vi "Meas Result Update View.vi"(8 "error in":errorcluster, 10 "gui refs":T15, 11 "meas":T3 {"swp cfg"."f list"."bias" format="%#_3p"; "swp cfg"."f list"."level" format="%#_3p"; "swp cfg"."f list"."fs [Hz]" format="%#_5p"; "swp cfg"."f list"."time [s]" format="%#_3p"; "swp cfg"."f list"."f/fs" format="%#_3p"; "swp cfg"."f list"."periods" format="%#_3f"; "swp cfg"."f list"."f [Hz]" format="%#_5p"}) -> (0 "error out":errorcluster)   [LabVIEW 2013]
doc: "Update results view."
uses:
  Meas Result GUI References.ctl
  Meas Result Freq Format.ctl
  meas session.ctl
  Meas Sweep Config.ctl
  Meas Freq Info.ctl
  meas_swp_mode.ctl
  meas_sweep_flist_mode.ctl
  bridge/Bridge Session.ctl
  bridge/Bridge Type.ctl
  drivers/TWM client/TWM Session.ctl
  drivers/TWM client/TWM parameters.ctl
  source/Source Session.ctl
  source/Source Type.ctl
  drivers/AFG3101C/AFG3101C Session.ctl
  Meas Results.ctl
  bridge/Bridge Frequency Readings Data.ctl
  Meas Result Major Format.ctl
  Meas Result Deviation Format.ctl
  varilib/varilib.lvlib
panel:
  in  "mjr dev fmt":T1 caption="Enum"
  in  "mjr fmt":T2
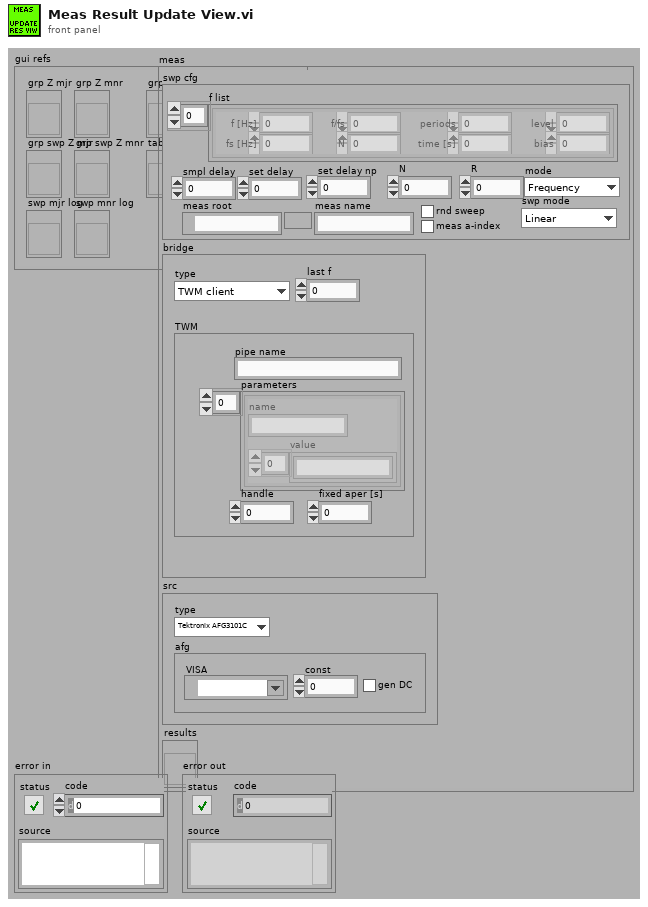
[diagram p1: front panel]
types:
  T1 = typedef "Meas Result Deviation Format.ctl" = enum16{"abs", "%", "ppm"}
  T2 = typedef "Meas Result Major Format.ctl" = enum16{"%_5p", "%_6p", "%_7p", "%_8p", "%_5f", "%_6f", "%_7f", "%_8f"}
  T3 = typedef "meas session.ctl" = cluster{"swp cfg":T4, "bridge":T8, "src":T12, "results":refnum<vi>}
  T4 = typedef "Meas Sweep Config.ctl" = cluster{"N":i32, "R":i32, "f list":T5[], "smpl delay":dbl, "set delay":dbl, "set delay np":dbl, "meas root":path, "meas name":string, "meas a-index":bool, "rnd sweep":bool, "mode":T6, "swp mode":T7}
  T5 = typedef "Meas Freq Info.ctl" = cluster{"f [Hz]":dbl, "periods":dbl, "f/fs":dbl, "time [s]":dbl, "fs [Hz]":dbl, "N":i32, "level":dbl, "bias":dbl}
  T6 = typedef "meas_swp_mode.ctl" = enum16{"Frequency", "Level", "Bias"}
  T7 = typedef "meas_sweep_flist_mode.ctl" = enum16{"Linear", "Log10"}
  T8 = typedef "Bridge Session.ctl" = cluster{"type":T9, "TWM":T10, "last f":dbl}
  T9 = typedef "Bridge Type.ctl" = enum16{"TWM client", "dummy"}
  T10 = typedef "TWM Session.ctl" = cluster{"pipe name":string, "parameters":T11[], "handle":i32, "fixed aper [s]":dbl}
  T11 = typedef "TWM parameters.ctl" = cluster{"name":string, "value":string[]}
  T12 = typedef "Source Session.ctl" = cluster{"type":T13, "afg":T14}
  T13 = typedef "Source Type.ctl" = enum16{"Tektronix AFG3101C", "dummy"}
  T14 = typedef "AFG3101C Session.ctl" = cluster{"VISA":refnum<visa-resource-name>, "const":dbl, "gen DC":bool}
  T15 = typedef "Meas Result GUI References.ctl" = cluster{"grp Z mjr":refnum<vi>, "grp Z mnr":refnum<vi>, "grp swp Z mjr":refnum<vi>, "grp swp Z mnr":refnum<vi>, "swp mjr log":refnum<vi>, "swp mnr log":refnum<vi>, "grp ref":refnum<vi>, "tab swp":refnum<vi>, "mjr fmt":refnum<vi>, "mnr fmt":refnum<vi>, "mjr dev fmt":refnum<vi>, "mnr dev fmt":refnum<vi>, "res frq fmt":refnum<vi>}
  T16 = typedef "Meas Results.ctl" = cluster{"freqs":T17[], "locked":bool, "last fid":i32, "modified":bool, "mjr name":string, "mnr name":string}
  T17 = typedef "Bridge Frequency Readings Data.ctl" = cluster{"Udut":dbl[], "Iref":dbl[], "Udc":dbl[], "Idc":dbl[], "mjr":dbl[], "mnr":dbl[], "n":i32, "f [Hz]":dbl}
  T18 = typedef "Meas Results Sweep Data.ctl" = cluster{"Udut":dbl[], "Iref":dbl[], "Udc":dbl[], "Idc":dbl[], "mjr":dbl[], "mnr":dbl[], "f [Hz]":dbl[]}
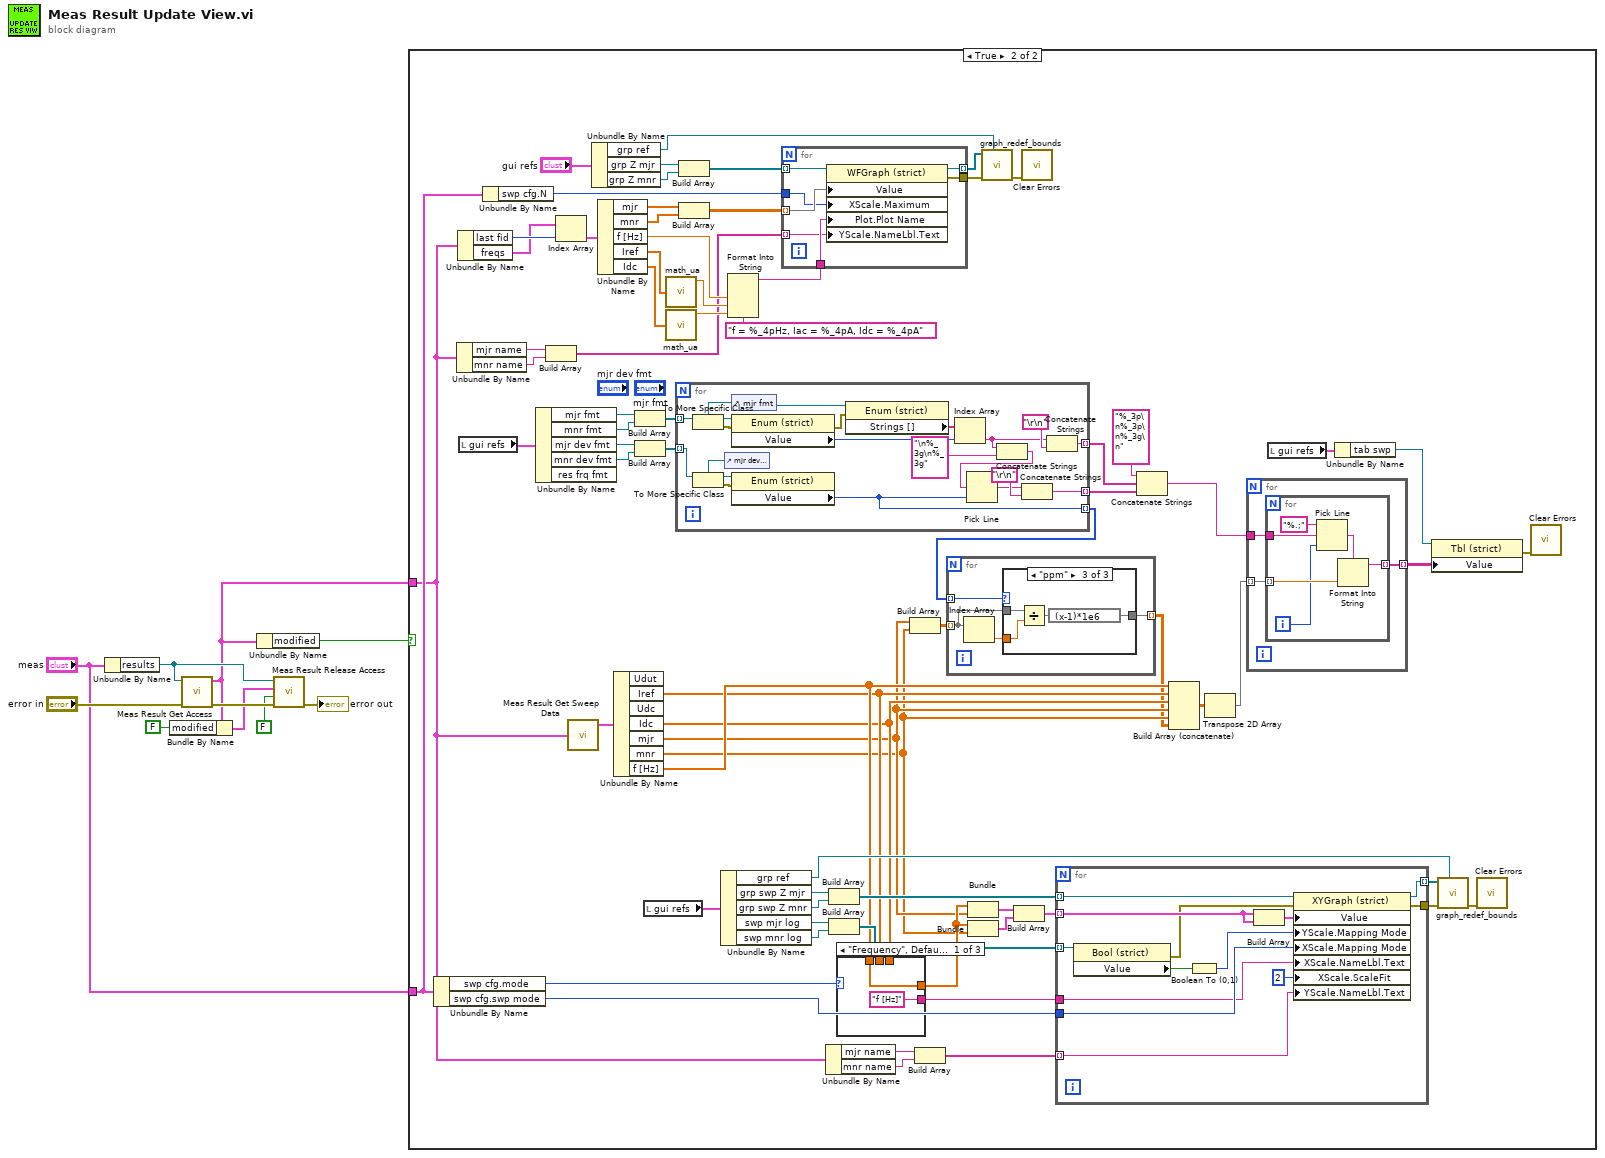
[diagram p0: block diagram]
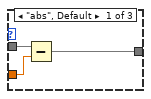
[diagram p3: hidden frame]
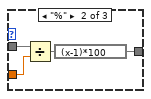
[diagram p4: hidden frame]
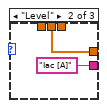
[diagram p5: hidden frame]
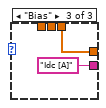
[diagram p6: hidden frame]
diagram:
  n1 = Unbundle By Name("meas") -> ("results"=w9:refnum<vi>)
  n2 = call "Meas Result Get Access.vi"("error in"="error in", "results ref"=w9) -> ("error out"=w10:errorcluster, "results data"=w2:T16)  [unwired: 8 in]
  n3 = Bundle By Name(cluster=w2, "modified"=FALSE) -> (w5:T16)
  n4 = Unbundle By Name(w2) -> ("modified"=w6:bool)
  n5 = call "Meas Result Release Access.vi"("error in"=w10, "Release only (True)"=FALSE, "results data in"=w5, "results ref"=w9) -> ("error out"=→"error out":errorcluster)  [unwired: 7 in]
  n6 = case shown="True" w6 {
    tunnel: w2 -> [_ w12]
    tunnel: "meas" -> [_ w46]
    frame False {
    }
    frame True {
      n7 = Unbundle By Name(w46) -> ("swp cfg.mode"=w67:T6, "swp cfg.swp mode"=w62:T7)
      n8 = Unbundle By Name(w12) -> ("mjr name"=w17:string, "mnr name"=w16:string)
      n9 = Unbundle By Name(w12) -> ("last fid"=w83:i32, "freqs"=w82:T17[])
      n10 = local read "gui refs"() -> (w33:T15)
      n11 = Unbundle By Name(w46) -> ("swp cfg.N"=w45:i32)
      n12 = Unbundle By Name(w33) -> ("mjr fmt"=w32:refnum<vi>, "mnr fmt"=w31:refnum<vi>, "mjr dev fmt"=w29:refnum<vi>, "mnr dev fmt"=w28:refnum<vi>)  [unwired: 1 out]
      n13 = Build Array(w17, w16) -> (w15:string[])
      n14 = Index Array(array=w82, index=w83) -> (element=w78:T17)
      n15 = call "Meas Result Get Sweep Data.vi"("result"=w12) -> ("data"=w37:T18)  [unwired: 2 out]
      n16 = Unbundle By Name("gui refs") -> ("grp ref"=w55:refnum<vi>, "grp Z mjr"=w81:refnum<vi>, "grp Z mnr"=w80:refnum<vi>)
      n17 = Unbundle By Name(w78) -> ("mjr"=w77:dbl[], "mnr"=w76:dbl[], "f [Hz]"=w39:dbl, "Iref"=w41:dbl[], "Idc"=w42:dbl[])
      n18 = Unbundle By Name(w37) -> ("Iref"=w35:dbl[], "Idc"=w34:dbl[], "mjr"=w22:dbl[], "mnr"=w21:dbl[], "f [Hz]"=w36:dbl[])  [unwired: 2 out]
      n19 = Build Array(w32, w31) -> (w30:refnum<vi>[])
      n20 = Build Array(w29, w28) -> (w27:refnum<vi>[])
      n21 = local read "gui refs"() -> (w74:T15)
      n22 = call "math_ua.vi"("x"=w41) -> ("mean(x)"=w40:dbl)  [unwired: 3 out]
      n23 = call "math_ua.vi"("x"=w42) -> ("mean(x)"=w43:dbl)  [unwired: 3 out]
      n24 = for {
        tunnel: w30 -> [w119] mode=indexing
        tunnel: [w108] -> w26 mode=indexing
        tunnel: w27 -> [w111] mode=indexing
        tunnel: [w101] -> w23 mode=indexing
        tunnel: [w100] -> w19 mode=indexing
        n25 = control-ref of="mjr dev fmt"() -> (w109:refnum<vi>)
        n26 = To More Specific Class(target class=w109, reference=w111) -> (specific class reference=w112:refnum<vi>, error out=w113:errorcluster)  [unwired: 1 in]
        n27 = control-ref of="mjr fmt"() -> (w110:refnum<vi>)
        n28 = To More Specific Class(target class=w110, reference=w119) -> (specific class reference=w118:refnum<vi>, error out=w117:errorcluster)  [unwired: 1 in]
        n29 = property class="Enum (strict)"(reference=w118, error in=w117) -> (error out=w114:errorcluster, "Value"=w115:T2)  [unwired: 1 out]
        n30 = property class="Enum (strict)"(reference=w112, error in=w113) -> ("Value"=w100:T1)  [unwired: 2 out]
        n31 = property class="Enum (strict)"(reference=w110, error in=w114) -> ("Strings []"=w116:string[])  [unwired: 2 out]
        n32 = Index Array(array=w116, index=w115) -> (element=w105:string)
        n33 = Concatenate Strings(w105, "\n%_3g\n%_3g") -> (w103:string)
        n34 = Pick Line(multi-line string=w103, line index=w100) -> (output string=w102:string)  [unwired: 1 in]
        n35 = Concatenate Strings(w102, "\r\n") -> (w101:string)
        n36 = Concatenate Strings(w105, "\r\n") -> (w108:string)
      }
      n37 = Build Array(w81, w80) -> (w79:refnum<vi>[])
      n38 = Build Array(w77, w76) -> (w75:dbl[][])
      n39 = Unbundle By Name(w74) -> ("grp ref"=w54:refnum<vi>, "grp swp Z mjr"=w73:refnum<vi>, "grp swp Z mnr"=w72:refnum<vi>, "swp mjr log"=w65:refnum<vi>, "swp mnr log"=w64:refnum<vi>)
      n40 = Format Into String(format string="f = %_4pHz, Iac = %_4pA, Idc = %_4pA", w39, w40, w43) -> (resulting string=w38:string)  [unwired: 2 in, 1 out]
      n41 = for {
        tunnel: w79 -> [w154] mode=indexing
        tunnel: w75 -> [w153] mode=indexing
        tunnel: [w152] -> w61
        tunnel: [w151] -> w59 mode=indexing
        tunnel: w45 -> [w150]
        tunnel: w38 -> [w149]
        tunnel: w15 -> [w148] mode=indexing
        n42 = property class="WFGraph (strict)"(reference=w154, "Value"=w153, "XScale.Maximum"=w150, "Plot.Plot Name"=w149, "YScale.NameLbl.Text"=w148) -> (reference out=w151:refnum<vi>, error out=w152:errorcluster)  [unwired: 1 in]
      }
      n43 = Unbundle By Name(w12) -> ("mjr name"=w13:string, "mnr name"=w14:string)
      n44 = Build Array(w73, w72) -> (w71:refnum<vi>[])
      n45 = Build Array(w65, w64) -> (w63:refnum<vi>[])
      n46 = case shown="\"Frequency\", Default" w67 {
        tunnel: [w130 w132 w134] -> w66
        tunnel: w36 -> [w130 _ _]
        tunnel: w35 -> [_ w132 _]
        tunnel: w34 -> [_ _ w134]
        tunnel: ["f [Hz]" "Iac [A]" "Idc [A]"] -> w53
        frame "Frequency", Default {
        }
        frame "Level" {
        }
        frame "Bias" {
        }
      }
      n47 = Build Array(w22, w21) -> (w20:dbl[][])
      n48 = Build Array(w13, w14) -> (w11:string[])
      n49 = for {
        tunnel: w20 -> [w86] mode=indexing
        tunnel: w19 -> [w88] mode=indexing
        tunnel: [w85] -> w18 mode=indexing
        n50 = Index Array(array=w86) -> (element=w87:dbl)  [unwired: 1 in]
        n51 = case shown="\"ppm\"" w88 {
          tunnel: w87 -> [w90 w93 w97]
          tunnel: w86 -> [w91 w94 w98]
          tunnel: [w89 w92 w96] -> w85
          frame "abs", Default {
            n52 = Subtract(x=w91, y=w90) -> (x-y=w89:dbl[])
          }
          frame "%" {
            n53 = Divide(x=w94, y=w93) -> (x/y=w95:dbl[])
            n54 = expression code="(x-1)*100"(w95) -> (w92:dbl[])
          }
          frame "ppm" {
            n55 = Divide(x=w98, y=w97) -> (x/y=w99:dbl[])
            n56 = expression code="(x-1)*1e6"(w99) -> (w96:dbl[])
          }
        }
      }
      n57 = Bundle("Idc"=w66, "mjr"=w22) -> (w70:cluster{"Idc":dbl[], "mjr":dbl[]})  [unwired: 1 in]
      n58 = Bundle("Idc"=w66, "mnr"=w21) -> (w69:cluster{"Idc":dbl[], "mnr":dbl[]})  [unwired: 1 in]
      n59 = call "graph_redef_bounds.vi"("grp ref pos"=w55, "error in"=w61, "graph refs in"=w59) -> ("error out"=w60:errorcluster)  [unwired: 7 in, 1 out]
      n60 = Build Array(w70, w69) -> (w68:cluster{"Idc":dbl[], "mnr":dbl[]}[])
      n61 = call <vilib>:"Clear Errors.vi"("error in (no error)"=w60) -> ()  [unwired: 6 in, 1 out]
      n62 = for {
        tunnel: w71 -> [w147] mode=indexing
        tunnel: w68 -> [w145] mode=indexing
        tunnel: w63 -> [w144] mode=indexing
        tunnel: w62 -> [w140]
        tunnel: [w139] -> w58
        tunnel: [w138] -> w57 mode=indexing
        tunnel: w53 -> [w137]
        tunnel: w11 -> [w135] mode=indexing
        n63 = property class="Bool (strict)"(reference=w144) -> (error out=w143:errorcluster, "Value"=w142:bool)  [unwired: 1 in, 1 out]
        n64 = Boolean To (0,1)(Boolean=w142) -> (0, 1=w141:i16)
        n65 = Build Array(w145, w145) -> (w146:cluster{"Idc":dbl[], "mnr":dbl[]}[])
        n66 = property class="XYGraph (strict)"(reference=w147, error in=w143, "Value"=w146, "YScale.Mapping Mode"=w141, "XScale.Mapping Mode"=w140, "XScale.NameLbl.Text"=w137, "XScale.ScaleFit"=u8 2 ("X Scale.Scale Fit"), "YScale.NameLbl.Text"=w135) -> (reference out=w138:refnum<vi>, error out=w139:errorcluster)
      }
      n67 = Concatenate Strings("%_3p\n%_3p\n%_3g\n", w26, w23) -> (w24:string)
      n68 = Build Array (concatenate)(w36, w35, w34, w22, w21, w18) -> (w52:dbl[][])
      n69 = Transpose 2D Array(2D array=w52) -> (transposed array=w51:dbl[][])
      n70 = for {
        tunnel: w24 -> [w122]
        tunnel: w51 -> [w121] mode=indexing
        tunnel: [w120] -> w48 mode=indexing
        n71 = for {
          tunnel: w122 -> [w128]
          tunnel: [w125] -> w120 mode=indexing
          tunnel: w121 -> [w124] mode=indexing
          i -> [w123]
          n72 = Pick Line(string ("")="%.;", multi-line string=w128, line index=w123) -> (output string=w127:string)
          n73 = Format Into String(format string=w127, w124) -> (resulting string=w125:string)  [unwired: 2 in, 1 out]
        }
      }
      n74 = local read "gui refs"() -> (w50:T15)
      n75 = Unbundle By Name(w50) -> ("tab swp"=w49:refnum<vi>)
      n76 = property class="Tbl (strict)"(reference=w49, "Value"=w48) -> (error out=w47:errorcluster)  [unwired: 1 in, 1 out]
      n77 = call "graph_redef_bounds.vi"("grp ref pos"=w54, "error in"=w58, "graph refs in"=w57) -> ("error out"=w56:errorcluster)  [unwired: 7 in, 1 out]
      n78 = call <vilib>:"Clear Errors.vi"("error in (no error)"=w56) -> ()  [unwired: 6 in, 1 out]
      n79 = call <vilib>:"Clear Errors.vi"("error in (no error)"=w47) -> ()  [unwired: 6 in, 1 out]
    }
  }
